vi "OpenShortDeEmbed_Write.vi"() -> ()   [LabVIEW 2017]
panel:
  out "error out":errorcluster
  in  "error in (no error)":errorcluster
  out "Intrinsic DUT S-parameter Trace Array":T1(array[cluster])=[{"Freq (Hz)"=5000000.0, "S-parameter Array"=[[0.0+0.0i, 1.0+0.0i], [1.0+0.0i, 0.0+0.0i]]}] {"Freq (Hz)" format="%.2e"; "S-parameter Array" format="%.3f"}
  in  "Short S-parameter File":path
  in  "Open S-parameter File":path
  in  "Extrinsic S-parameter File":path
  # "Performs Open-Short De-Embedding on 'extrinsic' S-parameters and Writes Result File\n\nAppends _OSdeembed to filename and puts in same folder"
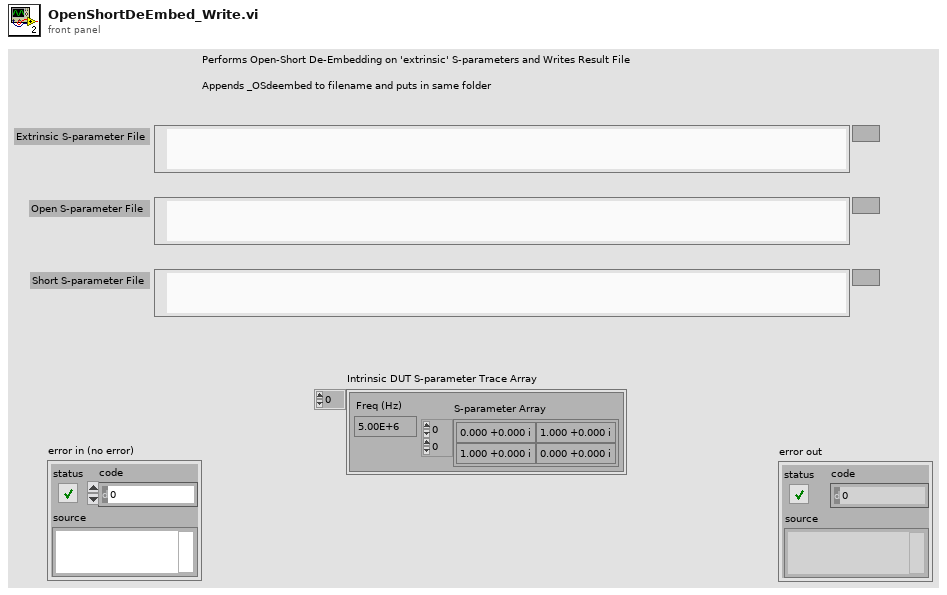
[diagram p1: front panel]
types:
  T1 = cluster{"Freq (Hz)":dbl, "S-parameter Array":csg[][]}[]
  T2 = cluster{"Comments":string, "Ref Impedance":u16, "Trace Array":cluster{"Freq (Hz)":dbl, "S-parameter Array":cdb[][]}[]}
  T3 = cluster{"Freq (Hz)":dbl, "S-parameter Array":cdb[][]}[]
  T4 = cluster{string, "Ref Impedance":u16, "Intrinsic DUT S-parameter Trace Array":cluster{"Freq (Hz)":dbl, "S-parameter Array":csg[][]}[]}
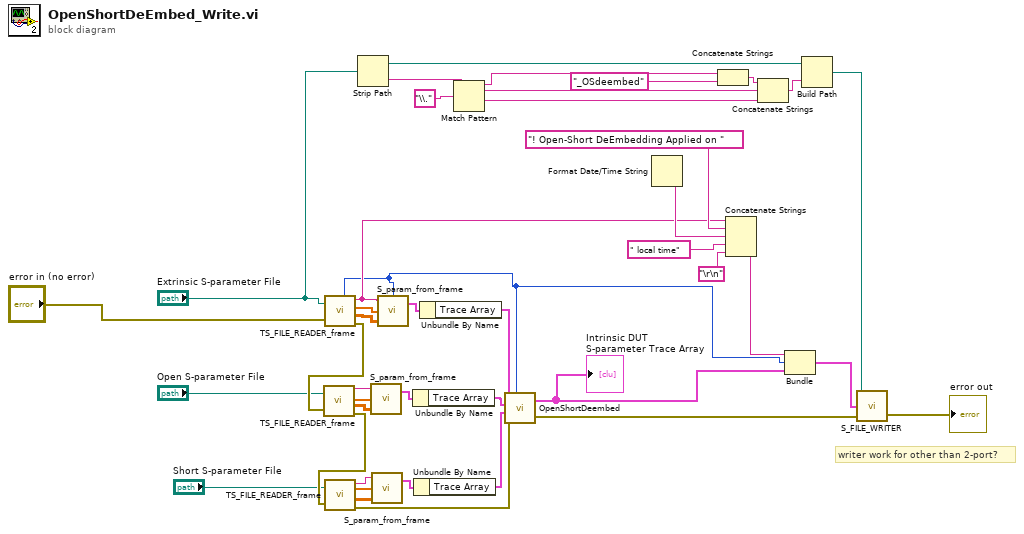
[diagram p0: block diagram]
diagram:
  # "writer work for other than 2-port?"
  n1 = call "TS_FILE_READER_frame.VI"("error in (no error)"="error in (no error)", "File"="Extrinsic S-parameter File") -> ("error out"=w42:errorcluster, "S-parameter Array"=w21:cdb[][], "Frequency Array"=w20:dbl[], "Comments"=w22:string, "Ref Impedance"=w2:u16)
  n2 = call "TS_FILE_READER_frame.VI"("error in (no error)"=w42, "File"="Open S-parameter File") -> ("error out"=w41:errorcluster, "S-parameter Array"=w13:cdb[][], "Frequency Array"=w14:dbl[], "Comments"=w15:string)  [unwired: 1 out]
  n3 = call "TS_FILE_READER_frame.VI"("error in (no error)"=w41, "File"="Short S-parameter File") -> ("error out"=w40:errorcluster, "S-parameter Array"=w6:cdb[][], "Frequency Array"=w7:dbl[], "Comments"=w8:string)  [unwired: 1 out]
  n4 = Strip Path(path="Extrinsic S-parameter File") -> (stripped path=w32:path, name=w30:string)
  n5 = call "S_param_from_frame.VI"("S-parameter Array"=w13, "Frequencies (Hz)"=w14, "Comments"=w15) -> ("Data Output"=w11:T2)  [unwired: 2 in]
  n6 = call "S_param_from_frame.VI"("S-parameter Array"=w6, "Frequencies (Hz)"=w7, "Comments"=w8) -> ("Data Output"=w10:T2)  [unwired: 2 in]
  n7 = call "S_param_from_frame.VI"("Ref Impedance"=w2, "S-parameter Array"=w21, "Frequencies (Hz)"=w20, "Comments"=w22) -> ("Data Output"=w17:T2)  [unwired: 1 in]
  n8 = Unbundle By Name(w11) -> ("Trace Array"=w12:T3)
  n9 = Unbundle By Name(w10) -> ("Trace Array"=w9:T3)
  n10 = Unbundle By Name(w17) -> ("Trace Array"=w16:T3)
  n11 = Match Pattern(string=w30, regular expression="\\.") -> (before substring=w24:string, match substring=w26:string, after substring=w27:string)  [unwired: 1 in, 1 out]
  n12 = call "OpenShortDeembed.vi"("Extrinsic DUT S-parameter Trace Array"=w16, "Open S-parameter Trace Array"=w12, "Short S-parameter Trace Array"=w9, "error in (no error)"=w40, "Reference Impedance"=w2) -> ("Intrinsic DUT S-parameter Trace Array"=w3:T1, "error out"=w38:errorcluster)
  "Intrinsic DUT S-parameter Trace Array" <- w3
  n13 = Format Date/Time String() -> (date/time string=w34:string)  [unwired: 3 in]
  n14 = Concatenate Strings(w24, "_OSdeembed") -> (w25:string)
  n15 = Concatenate Strings(w22, "! Open-Short DeEmbedding Applied on ", w34, " local time", "\r\n") -> (w4:string)
  n16 = Concatenate Strings(w25, w26, w27) -> (w28:string)
  n17 = Bundle(w4, "Ref Impedance"=w2, "Intrinsic DUT S-parameter Trace Array"=w3) -> (w1:T4)  [unwired: 1 in]
  n18 = Build Path(base path=w32, name or relative path=w28) -> (appended path=w31:path)
  n19 = call "S_FILE_WRITER.VI"("error in (no error)"=w38, "Data Input"=w1, "Input Path"=w31) -> ("error out"=→"error out":errorcluster)  [unwired: 1 in, 1 out]
